vi "Execute Line Test and Control.vi"(5 "Right Encoder RefNum":string, 6 "Left Encoder RefNum":string, 7 "Right Sensor RefNum":string, 8 "Left Sensor RefNum":string) -> (0 "Right Encoder":dbl, 1 "Left Encoder":dbl, 2 "Y-Axis To Drive":dbl, 3 "X-Axis To Drive":dbl)   [LabVIEW 2013]
panel:
  out "Right":bool
  out "Left":bool
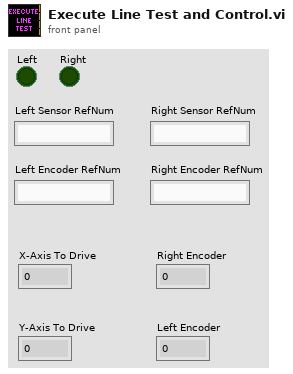
[diagram p1: front panel]
types:
  T1 = typedef "WPI_DigitalInputDevRef.ctl" = cluster{"DevStatus":errorcluster, "DIO Channel":T2, "Digital Module":T3}
  T2 = typedef "FPGA_DIOChannel.ctl" = enum8{"DIO 1", "DIO 2", "DIO 3", "DIO 4", "DIO 5", "DIO 6", "DIO 7", "DIO 8", "DIO 9", "DIO 10", "DIO 11", "DIO 12", "DIO 13", "DIO 14", "Invalid"}
  T3 = typedef "FPGA_TypedefDigitalModule.ctl" = enum16{"Digital Module 1", "Digital Module 2"}
  T4 = typedef "WPI_EncoderDevRef.ctl" = cluster{"DevStatus":errorcluster, "EncoderIndex":T5, "CounterIndex":T6, "DistancePerCount":dbl, "Decoding Type":T7}
  T5 = typedef "FPGA_EncoderIdx.ctl" = enum8{"Enc 0", "Enc 1", "Enc 2", "Enc 3", "Invalid"}
  T6 = typedef "FPGA_CounterCtrSystemIndex.ctl" = enum8{"Ctr 0", "Ctr 1", "Ctr 2", "Ctr 3", "Ctr 4", "Ctr 5", "Ctr 6", "Ctr 7", "Invalid"}
  T7 = typedef "WPI_EncoderType.ctl" = enum16{"1x", "2x", "4x"}
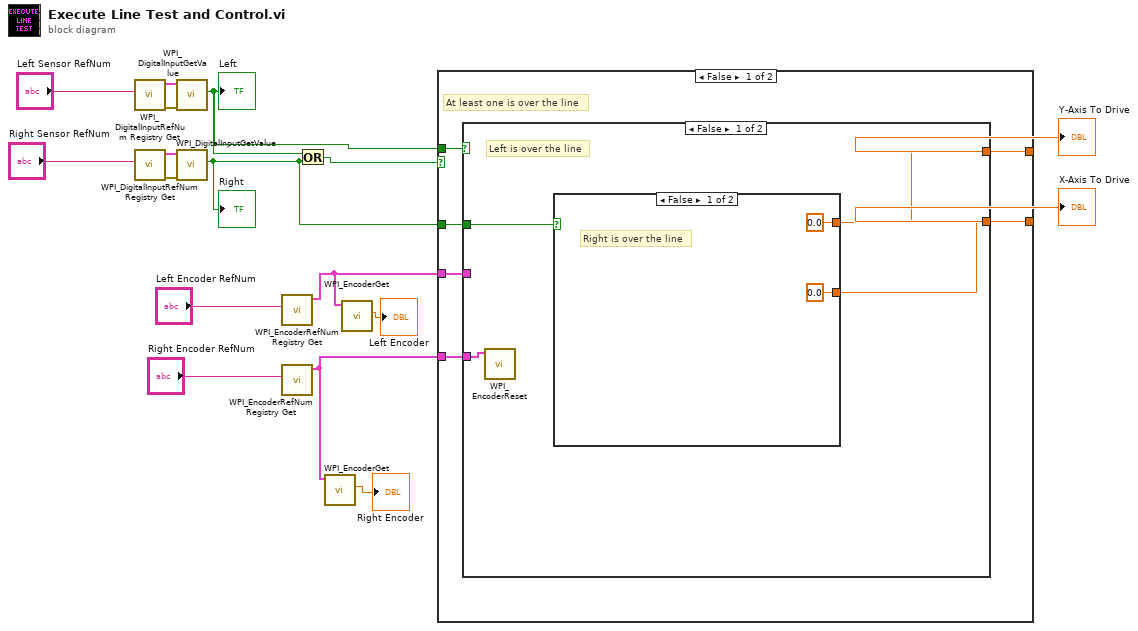
[diagram p0: block diagram]
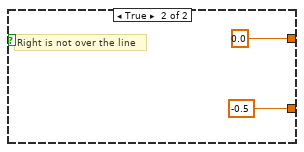
[diagram p2: hidden frame]
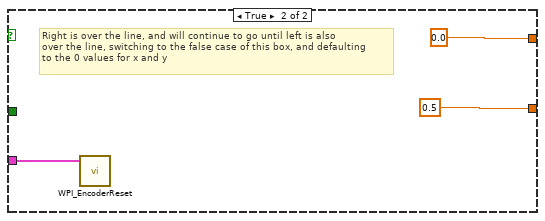
[diagram p3: hidden frame]
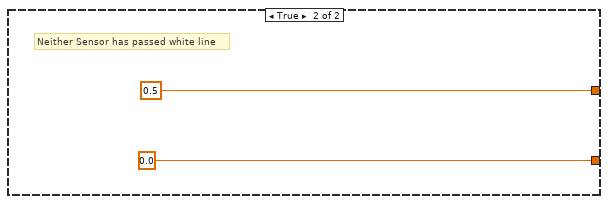
[diagram p4: hidden frame]
diagram:
  n1 = call <vilib>:"WPI_DigitalInputRefNum Registry Get.vi"("refnum name"="Left Sensor RefNum") -> ("error out"=w12:errorcluster, "DigitalInputDevRef"=w15:T1)  [unwired: 9 in]
  n2 = call <vilib>:"WPI_DigitalInputRefNum Registry Get.vi"("refnum name"="Right Sensor RefNum") -> ("error out"=w13:errorcluster, "DigitalInputDevRef"=w14:T1)  [unwired: 9 in]
  n3 = call <vilib>:"WPI_DigitalInputGetValue.vi"("error in (no error)"=w12, "DigitalInputDevRef"=w15) -> ("Value"=w10:bool)  [unwired: 7 in, 2 out]
  "Left" <- w10
  n4 = call <vilib>:"WPI_DigitalInputGetValue.vi"("error in (no error)"=w13, "DigitalInputDevRef"=w14) -> ("Value"=w5:bool)  [unwired: 7 in, 2 out]
  "Right" <- w5
  n5 = call <vilib>:"WPI_EncoderRefNum Registry Get.vi"("refnum name"="Left Encoder RefNum") -> ("EncoderDevRef"=w4:T4)  [unwired: 9 in, 1 out]
  n6 = call <vilib>:"WPI_EncoderRefNum Registry Get.vi"("refnum name"="Right Encoder RefNum") -> ("EncoderDevRef"=w3:T4)  [unwired: 9 in, 1 out]
  n7 = Or(x=w10, y=w5) -> (x .or. y?=w11:bool)
  n8 = call <vilib>:"WPI_EncoderGet.vi"("EncoderDevRef"=w3) -> ("Distance"=→"Right Encoder":dbl)  [unwired: 5 in, 5 out]
  n9 = call <vilib>:"WPI_EncoderGet.vi"("EncoderDevRef"=w4) -> ("Distance"=→"Left Encoder":dbl)  [unwired: 5 in, 5 out]
  n10 = case shown="False" w11 {
    tunnel: w10 -> [w23 _]
    tunnel: [w22 0.0 ("X-Axis To Drive")] -> w9
    tunnel: [w21 0.5 ("Y-Axis To Drive")] -> w8
    tunnel: w4 -> [w20 _]
    tunnel: w3 -> [w19 _]
    tunnel: w5 -> [w18 _]
    frame False {
      # "At least one is over the line"
      n11 = case shown="False" w23 {
        tunnel: [w25 0.5 ("X-Axis To Drive")] -> w22
        tunnel: [w26 0.0 ("X-Axis To Drive")] -> w21
        tunnel: w20 -> [_ w32]
        tunnel: w19 -> [w24 _]
        tunnel: w18 -> [w27 _]
        frame False {
          # "Left is over the line"
          n12 = call <vilib>:"WPI_EncoderReset.vi"("EncoderDevRef"=w24) -> ()  [unwired: 9 in, 2 out]
          n13 = case shown="False" w27 {
            tunnel: [0.0 ("X-Axis To Drive") 0.0 ("X-Axis To Drive")] -> w26
            tunnel: [0.0 ("X-Axis To Drive") -0.5 ("X-Axis To Drive")] -> w25
            frame False {
              # "Right is over the line"
            }
            frame True {
              # "Right is not over the line"
            }
          }
        }
        frame True {
          # "Right is over the line, and will continue to go until left is also\nover the line, switching to the false case of this box, and defaulting\nto the 0 values for x and y"
          n14 = call <vilib>:"WPI_EncoderReset.vi"("EncoderDevRef"=w32) -> ()  [unwired: 9 in, 2 out]
        }
      }
    }
    frame True {
      # "Neither Sensor has passed white line"
    }
  }
  "X-Axis To Drive" <- w9
  "Y-Axis To Drive" <- w8
